vi "信息框（标题、文本）.vi"(8 "错误输入（无错误）":errorcluster, 9 "buttons":i32(ring) items=["OK", "OKCancel", "AbortRetryIgnore", "YesNoCancel", "YesNo", "RetryCancel"], 10 "caption":string, 11 "text":string) -> (0 "错误输出":errorcluster)   [LabVIEW 2011]
uses:
  System.Windows.Forms
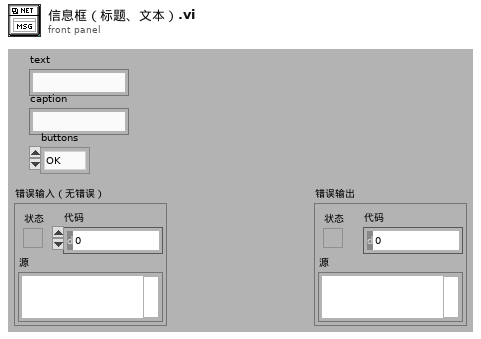
[diagram p1: front panel]
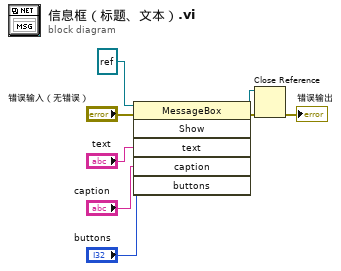
[diagram p0: block diagram]
diagram:
  n1 = invoke class="MessageBox" method="Show"(reference=refnum<k24> refnum, error in="错误输入（无错误）", "text"="text", "caption"="caption", "buttons"="buttons") -> (reference out=w8:refnum<k24>, error out=w7:errorcluster)  [unwired: 1 in, 4 out]
  n2 = Close Reference(reference=w8, error in (no error)=w7) -> (error out=→"错误输出":errorcluster)
